vi "Initialize Global2.vi"(0 "System no.":i32=1 min=1 max=4 step=1, 5 "error in":errorcluster) -> (19 "error out":errorcluster)   [LabVIEW 2026]
doc: "This VI initializes Global2 (Array) according to the given system no."
uses:
  Global2 (Array).vi
panel:
  # "This vi initializes Global 2 (Array)\naccording to the given system no."
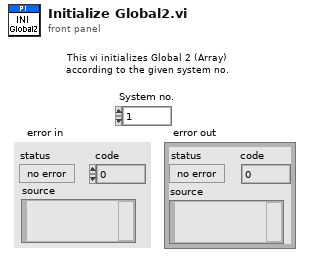
[diagram p1: front panel]
types:
  T1 = typedef "Controller names.ctl" = enum16{"None", "Analog", "C-702", "C-413", "C-414", "C-843", "C-843.PM", "C-844", "C-848", "C-865", "C-866", "C-867", "C-877", "C-880", "C-884", "C-885", "C-886", "C-887", "C-891", "E-135", "E-516", "E-517", "E-518", "E-709", "E-710", "E-712", "E-725", "E-727", "E-753", "E-754", "E-755", "E-761", "E-816", "E-861", "E-870", "E-871", "E-872", "E-873", "E-874", "F-206", "HydraPollux", "M-840", "M-850", "M-8X0", "Mercury", "Mercury_GCS", "PI_GCS2"}
  T2 = cluster{"Conn. axes":string[], "Controller name":T1}[]
  T3 = cluster{"Conn. axes":string[], "Controller name":T1}
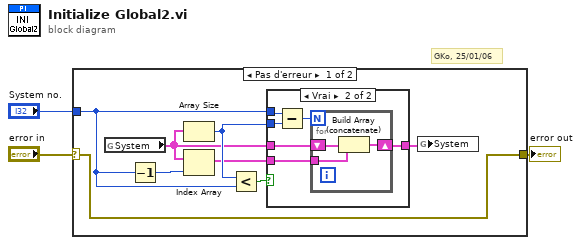
[diagram p0: block diagram]
diagram:
  # "GKo, 25/01/06"
  n1 = case shown="Pas d'erreur" "error in" {
    selector: "error in" -> [w4 w22]
    tunnel: "System no." -> [w10 _]
    tunnel: [w4 w22] -> w1
    frame No Error {
      n2 = global read "Global2 (Array).vi" "System"() -> (w6:T2)
      n3 = Decrement(x=w10) -> (x-1=w8:i32)
      n4 = Array Size(array=w6) -> (size(s)=w9:i32)
      n5 = Index Array(array=w6, index=w8) -> (element=w7:T3)
      n6 = Less?(x=w9, y=w10) -> (x < y?=w11:bool)
      n7 = case shown="Vrai" w11 {
        tunnel: w10 -> [_ w17]
        tunnel: w9 -> [_ w16]
        tunnel: w6 -> [w12 w15]
        tunnel: w7 -> [_ w14]
        tunnel: [w12 w13] -> w5
        frame False {
        }
        frame True {
          n8 = Subtract(x=w17, y=w16) -> (x-y=w18:i32)
          n9 = for {
            N: w18 -> [_]
            shift-right: [w21] -> w13
            shift-left: w15 -> [w20]
            tunnel: w14 -> [w19]
            n10 = Build Array (concatenate)(w20, w19) -> (w21:T2)
          }
        }
      }
      n11 = global write "Global2 (Array).vi" "System"(w5) -> ()
    }
    frame Error {
    }
  }
  "error out" <- w1
